vi "CAEN-PSM_1471.vi"() -> ()   [LabVIEW 2018]
doc: "This example shows how to configure the instrument's output voltage level, over current protection, and over voltage protection. The actual voltage level and actual current level are returned as well as whether over voltage protection (OVP) or over current protection (OCP) has been tripped."
uses:
  <vilib>/Utility/file.llb/Write To Spreadsheet File (string).vi
  <instrlib>/CAEN PSM/CAEN PSM.lvlib
panel:
  in  "Stop 1":bool
  in  "Tab Control":T1(tab)
  in  "Set":string[][](table)=[["", "", "", "", "", ""], ["", "", "", "", "", ""], ["", "", "", "", "", ""], ["", "", "", "", "", ""], ["", "", "", "", "", ""], ["", "", "", "", "", ""]]
  out "Monitor":string[][](table)
  in  "Ch (On/Off)":bool[](array[boolean])=[FALSE, FALSE, FALSE, FALSE, FALSE, FALSE, FALSE, FALSE]
  in  "Stop":bool
  in  "Comunication Port":refnum<visa-resource-name>="COM4"
  out "Channel Status":T2(array[cluster])
  in  "File name":string="Name"
  in  "Save":bool
  in  "Grid on/off":enum32{"Radio Selection 1", "Radio Selection 2"}(radio)=enum."Radio Selection 2"
  out "I CH0":T3(graph)
  out "V CH0":T4(graph)
  out "V Ch1":T4(graph)
  out "I CH1":T3(graph)
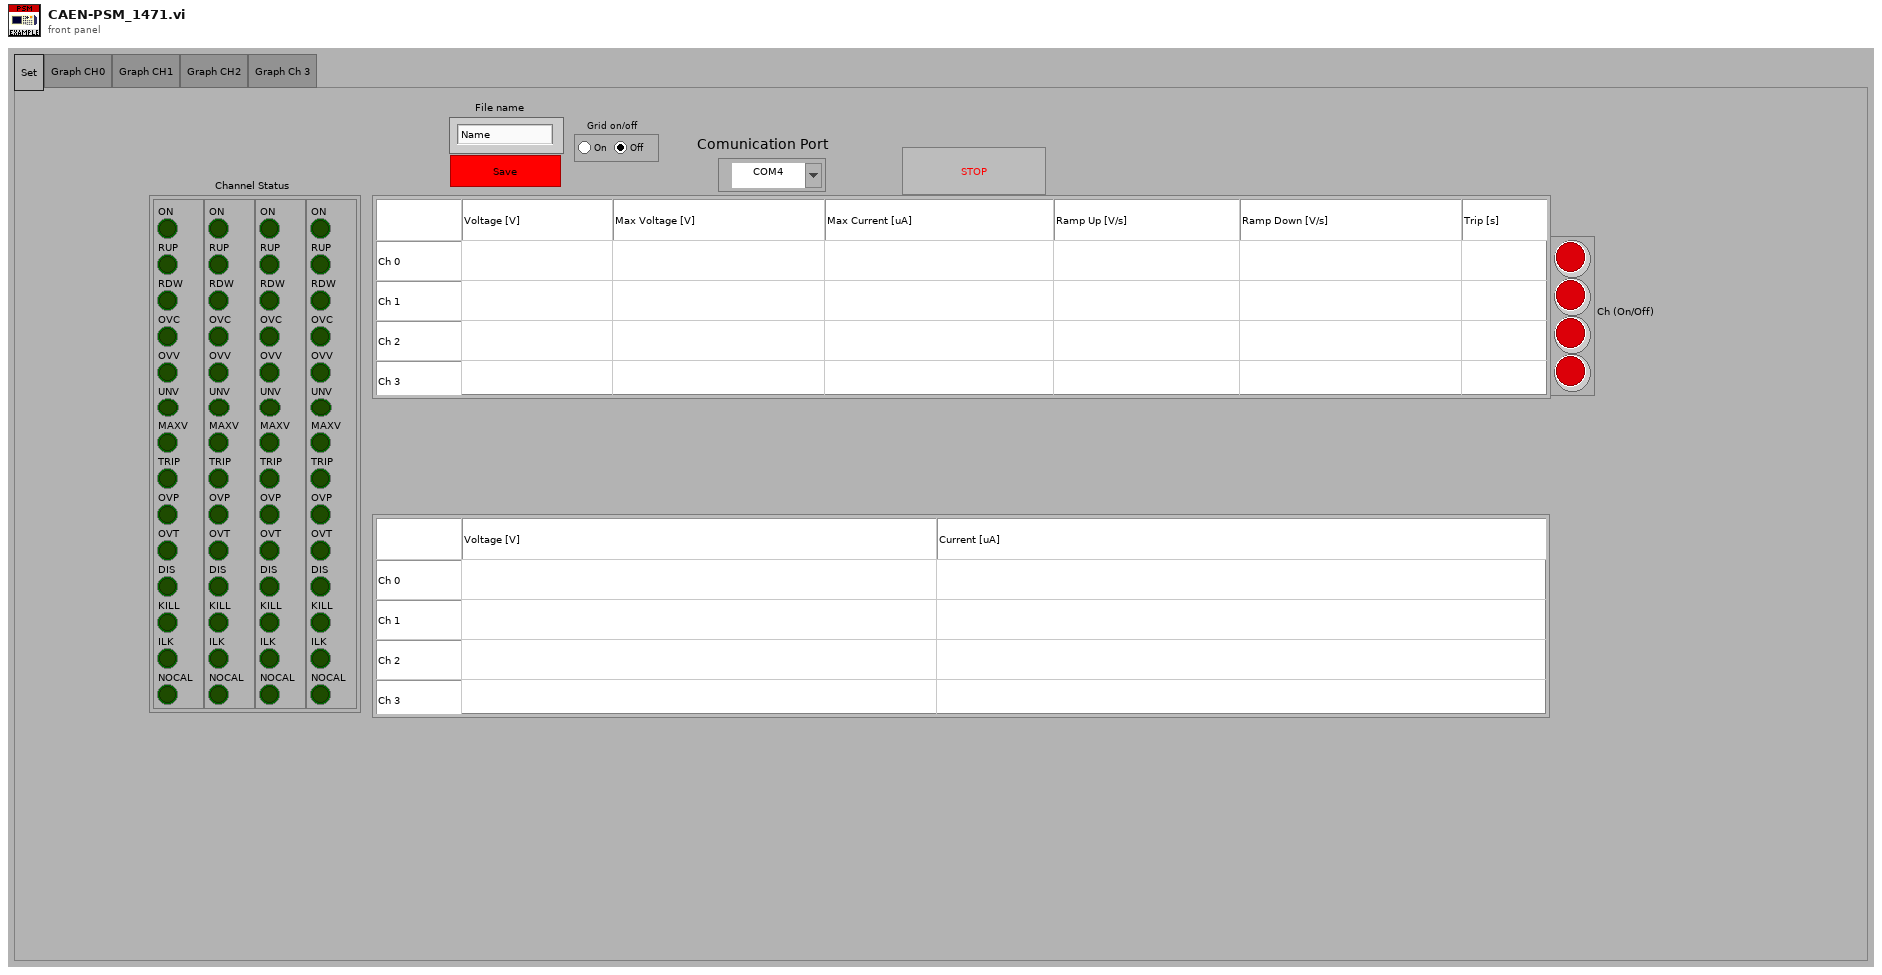
[diagram p1: front panel]
types:
  T1 = enum32{"Set", "Graph CH0", "Graph CH1", "Graph CH2", "Graph Ch 3"}
  T2 = cluster{"ON":bool, "RUP":bool, "RDW":bool, "OVC":bool, "OVV":bool, "UNV":bool, "MAXV":bool, "TRIP":bool, "OVP":bool, "OVT":bool, "DIS":bool, "KILL":bool, "ILK":bool, "NOCAL":bool}[]
  T3 = cluster{"seconds since 1Jan1904":timestamp, "IMon value":dbl}[]
  T4 = cluster{"seconds since 1Jan1904":timestamp, "VMon value":dbl}[]
  T5 = cluster{"Baud Rate":u32, "Parity":u16, "Data Bits":u16, "Stop Bits":u16, "Flow Control":u16}
  T6 = typedef "CAEN PSM.lvlib/BoardHandle.ctl" = cluster{"VISA resource name":refnum<visa-resource-name>, "Board address":u8, "NChannels":u8}
  T7 = cluster{"ON":bool, "RUP":bool, "RDW":bool, "OVC":bool, "OVV":bool, "UNV":bool, "MAXV":bool, "TRIP":bool, "OVP":bool, "OVT":bool, "DIS":bool, "KILL":bool, "ILK":bool, "NOCAL":bool}
  T8 = cluster{"seconds since 1Jan1904":timestamp, "VMon value":dbl}
  T9 = cluster{"seconds since 1Jan1904":timestamp, "IMon value":dbl}
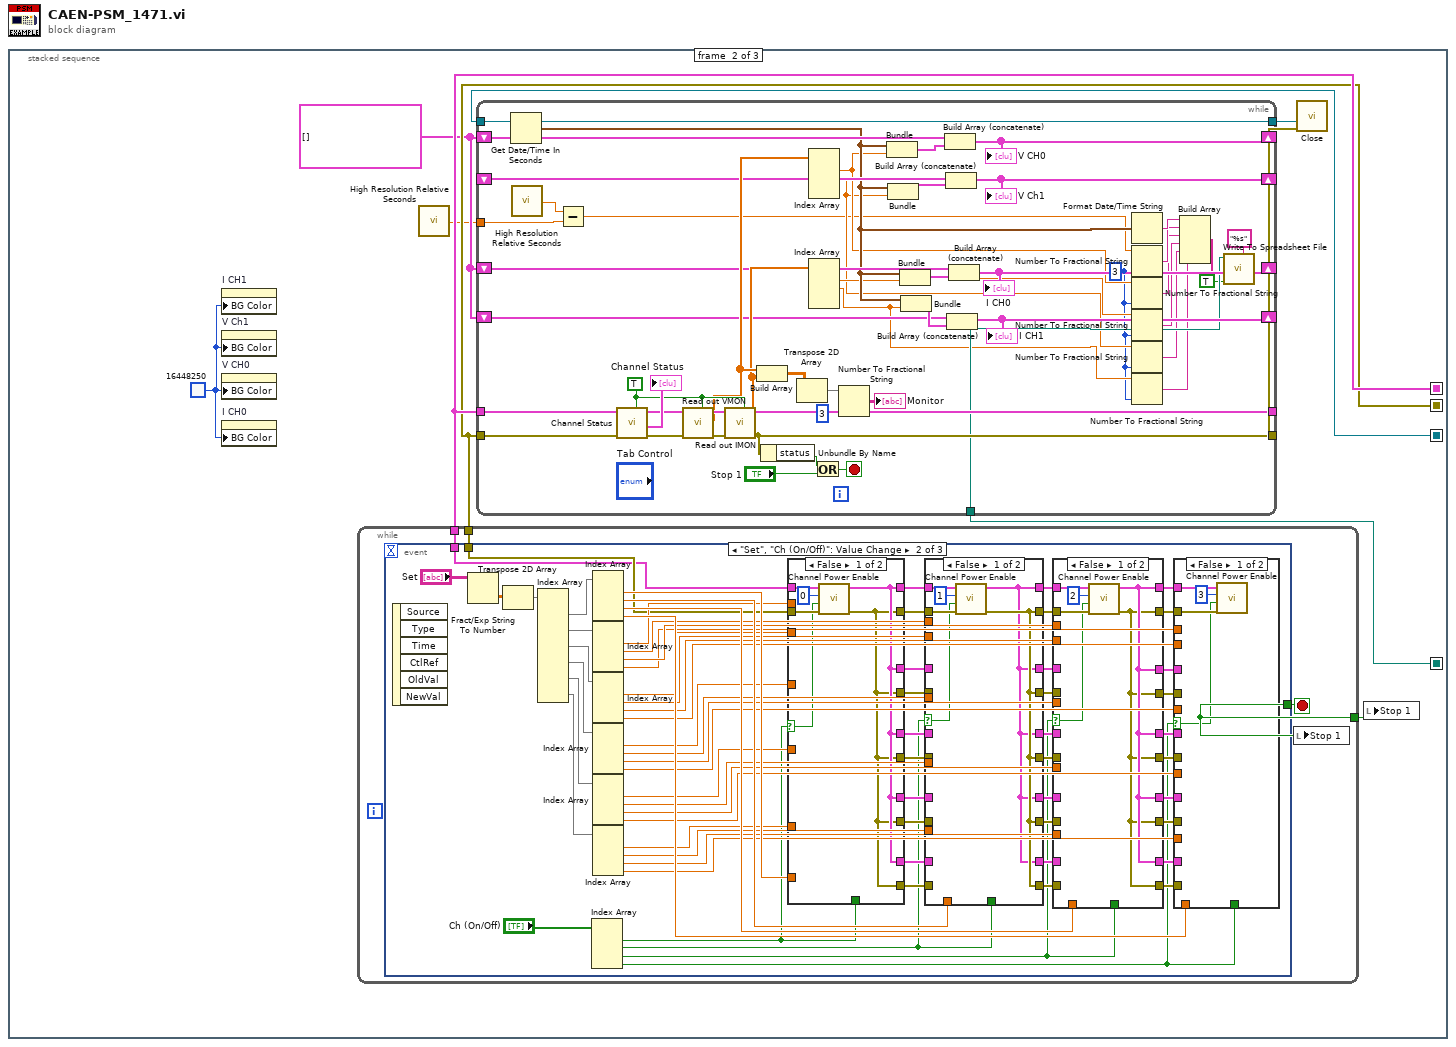
[diagram p0: block diagram]
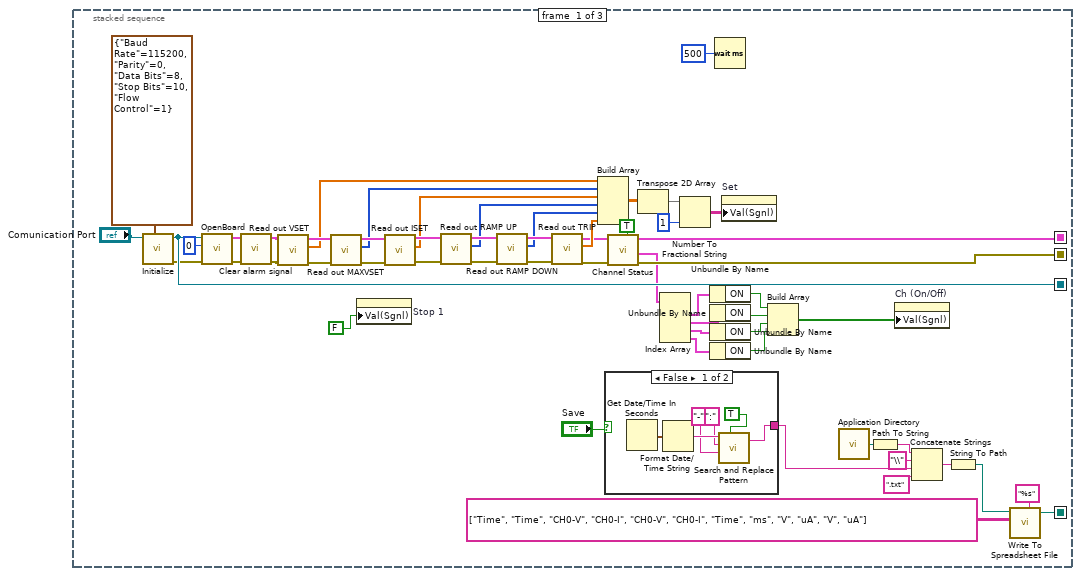
[diagram p2: hidden frame]
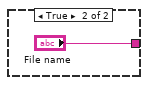
[diagram p3: hidden frame]
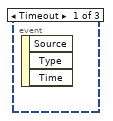
[diagram p4: hidden frame]
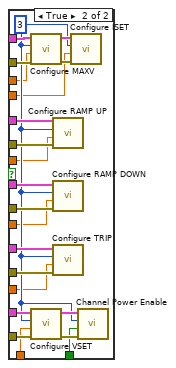
[diagram p5: hidden frame]
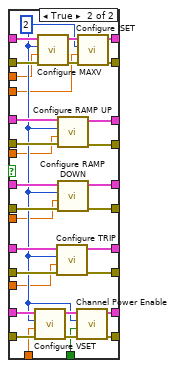
[diagram p6: hidden frame]
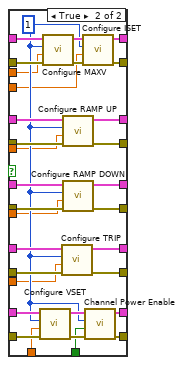
[diagram p7: hidden frame]
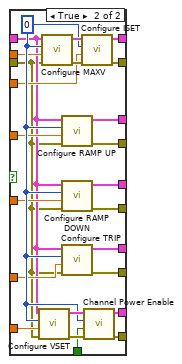
[diagram p8: hidden frame]
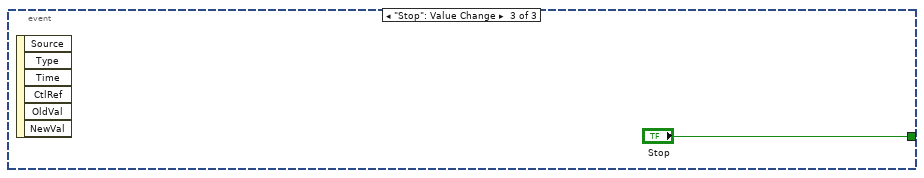
[diagram p9: hidden frame]
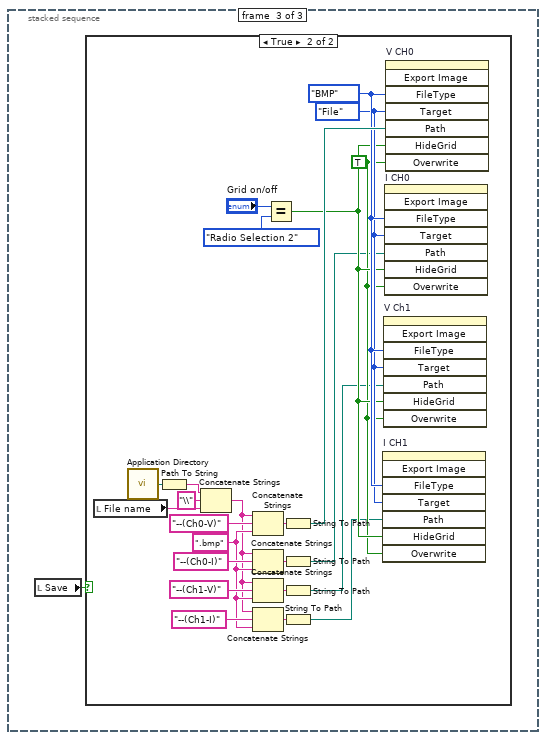
[diagram p10: hidden frame]
diagram:
  n1 = stacked-sequence {
    seq-local: [w56 _ _] -> [_ w71 _]
    seq-local: [w55 _ _] -> [_ w70 _]
    seq-local: [w57 _ _] -> [_ w74 _]
    seq-local: [w11 _ _] -> [_ w66 _]
    frame #0 {
      n2 = call <instrlib>:"Initialize.vi"("Serial Configuration"=T5 {"Baud Rate"=115200, "Parity"=0, "Data Bits"=8, "Stop Bits"=10, "Flow Control"=1}, "VISA resource name"="Comunication Port") -> ("error out"=w53:errorcluster, "VISA resource name out"=w57:refnum<visa-resource-name>)  [unwired: 8 in]
      n3 = call <instrlib>:"OpenBoard.vi"("error in (no error)"=w53, "Board Address"=u8 0, "VISA resource name"=w57) -> ("error out"=w51:errorcluster, "BoardHandle"=w50:T6)  [unwired: 7 in]
      n4 = call <instrlib>:"Clear alarm signal.vi"("error in (no error)"=w51, "BoardHandle"=w50) -> ("error out"=w37:errorcluster, "BoardHandle out"=w38:T6)  [unwired: 8 in]
      n5 = call <instrlib>:"Read out VSET.vi"("error in (no error)"=w37, "BoardHandle"=w38) -> ("error out"=w47:errorcluster, "Vset values (V)"=w33:dbl[], "BoardHandle out"=w48:T6)  [unwired: 6 in, 1 out]
      n6 = call <instrlib>:"Read out MAXVSET.vi"("error in (no error)"=w47, "BoardHandle"=w48) -> ("error out"=w45:errorcluster, "Voltage max values (V)"=w32:i32[], "BoardHandle out"=w46:T6)  [unwired: 6 in, 1 out]
      n7 = property on="Stop 1" class="Bool (strict)"("Val(Sgnl)"=FALSE ("Value (Signaling)")) -> ()  [unwired: 2 in, 2 out]
      n8 = call <instrlib>:"Read out ISET.vi"("error in (no error)"=w45, "BoardHandle"=w46) -> ("error out"=w43:errorcluster, "ISet values (uA)"=w31:dbl[], "BoardHandle out"=w44:T6)  [unwired: 6 in, 1 out]
      n9 = call <instrlib>:"Read out RAMP UP.vi"("error in (no error)"=w43, "BoardHandle"=w44) -> ("error out"=w41:errorcluster, "Ramp up values  (V/s)"=w30:i32[], "BoardHandle out"=w42:T6)  [unwired: 6 in, 1 out]
      n10 = call <instrlib>:"Read out RAMP DOWN.vi"("error in (no error)"=w41, "BoardHandle"=w42) -> ("error out"=w39:errorcluster, "Ramp down values  (V/s)"=w29:i32[], "BoardHandle out"=w40:T6)  [unwired: 6 in, 1 out]
      n11 = call <instrlib>:"Read out TRIP.vi"("error in (no error)"=w39, "BoardHandle"=w40) -> ("error out"=w24:errorcluster, "Trip values (s)"=w28:dbl[], "BoardHandle out"=w25:T6)  [unwired: 6 in, 1 out]
      n12 = Build Array(w33, w32, w31, w30, w29, w28) -> (w36:dbl[][])
      n13 = case shown="False" "Save" {
        tunnel: [w58 "File name"] -> w1
        frame False {
          n14 = Get Date/Time In Seconds() -> (seconds since 1Jan1904=w63:timestamp)
          n15 = Format Date/Time String(seconds (now)=w63) -> (date/time string=w62:string)  [unwired: 2 in]
          n16 = call <vilib>:"Search and Replace Pattern.vi"("string"=w62, "regular expression (\"\")"=":" ("regular expression (\"\")"), "replace string (\"\")"="-" ("replace string (\"\")"), "replace all? (F)"=TRUE) -> ("result string"=w58:string)  [unwired: 1 in, 1 out]
        }
        frame True {
        }
      }
      n17 = call <instrlib>:"Channel Status.vi"("All Channels (T)"=TRUE, "error in (no error)"=w24, "BoardHandle"=w25) -> ("error out"=w55:errorcluster, "Channel Status Array"=w23:T2, "BoardHandle out"=w56:T6)  [unwired: 6 in]
      n18 = Transpose 2D Array(2D array=w36) -> (transposed array=w35:dbl[][])
      n19 = Index Array(array=w23) -> (element #1=w22:T7, element #2=w21:T7, element #3=w20:T7, element #4=w19:T7)  [unwired: 4 in]
      n20 = Number To Fractional String(number=w35, precision (6)=i16 1) -> (F-format string=w27:string[][])  [unwired: 2 in]
      n21 = Unbundle By Name(w22) -> ("ON"=w18:bool)
      n22 = Unbundle By Name(w21) -> ("ON"=w17:bool)
      n23 = Unbundle By Name(w20) -> ("ON"=w16:bool)
      n24 = Unbundle By Name(w19) -> ("ON"=w15:bool)
      n25 = Wait (ms)(milliseconds to wait=u32 500) -> ()  [unwired: 1 out]
      n26 = property on="Set" class="Tbl (strict)"("Val(Sgnl)"=w27) -> ()  [unwired: 2 in, 2 out]
      n27 = Build Array(w18, w17, w16, w15) -> (w14:bool[])
      n28 = call <vilib>:"Application Directory.vi"() -> ("Application Directory"=w5:path)
      n29 = Path To String(path=w5) -> (string=w4:string)
      n30 = property on="Ch (On/Off)" class="Arr (strict)"("Val(Sgnl)"=w14) -> ()  [unwired: 2 in, 2 out]
      n31 = Concatenate Strings(w4, "\\" ("string"), w1, ".txt" ("string")) -> (w9:string)
      n32 = String To Path(string=w9) -> (path=w10:path)
      n33 = call-poly <vilib>:"Write To Spreadsheet File.vi"("format (%s)"="%s", "2D data"=string[][] [["Time", "Time", "CH0-V", "CH0-I", "CH0-V", "CH0-I"], ["Time", "ms", "V", "uA", "V", "uA"]], "file path (dialog if empty)"=w10) -> ("new file path (Not A Path if cancelled)"=w11:path)  [unwired: 5 in]
    }
    frame #1 {
      w67 = u32 16448250
      w68 = T4 []
      n34 = property on="I CH1" class="XYGraph (strict)"("BG Color"=w67) -> ()  [unwired: 2 in, 2 out]
      n35 = property on="V Ch1" class="XYGraph (strict)"("BG Color"=w67) -> ()  [unwired: 2 in, 2 out]
      n36 = property on="V CH0" class="XYGraph (strict)"("BG Color"=w67) -> ()  [unwired: 2 in, 2 out]
      n37 = property on="I CH0" class="XYGraph (strict)"("BG Color"=w67) -> ()  [unwired: 2 in, 2 out]
      n38 = while {
        tunnel: w71 -> [w77]
        tunnel: w70 -> [w76]
        tunnel: [w75] -> w69
        stop <- w75 stop-if-true
        n39 = event shown="[1] \"Set\", \"Ch (On/Off)\": Value Change" {
          selector: _ -> [_ _ _]
          dyn-events: _ -> [_ _ _]
          timeout: _ -> [_ _ _]
          tunnel: [_ _ "Stop"] -> w75
          tunnel: w77 -> [_ w82 _]
          tunnel: w76 -> [_ w83 _]
          event Timeout {
            n40 = event-data() -> ()  [unwired: 1 in, 3 out]
          }
          event "Set", "Ch (On/Off)": Value Change {
            n41 = event-data() -> ()  [unwired: 1 in, 6 out]
            n42 = Fract/Exp String To Number(string="Set") -> (number=w117:dbl[][])  [unwired: 3 in, 1 out]
            n43 = Transpose 2D Array(2D array=w117) -> (transposed array=w116:dbl[][])
            n44 = Index Array(array=w116) -> (element #1=w115:dbl[], element #2=w114:dbl[], element #3=w113:dbl[], element #4=w112:dbl[], element #5=w111:dbl[], element #6=w110:dbl[])  [unwired: 12 in]
            n45 = Index Array(array="Ch (On/Off)") -> (element #1=w81:bool, element #2=w80:bool, element #3=w79:bool, element #4=w78:bool)  [unwired: 4 in]
            n46 = Index Array(array=w115) -> (element #1=w109:dbl, element #2=w108:dbl, element #3=w107:dbl, element #4=w106:dbl)  [unwired: 4 in]
            n47 = Index Array(array=w114) -> (element #1=w105:dbl, element #2=w104:dbl, element #3=w103:dbl, element #4=w102:dbl)  [unwired: 4 in]
            n48 = Index Array(array=w113) -> (element #1=w101:dbl, element #2=w100:dbl, element #3=w99:dbl, element #4=w98:dbl)  [unwired: 4 in]
            n49 = Index Array(array=w112) -> (element #1=w97:dbl, element #2=w96:dbl, element #3=w95:dbl, element #4=w94:dbl)  [unwired: 4 in]
            n50 = Index Array(array=w111) -> (element #1=w93:dbl, element #2=w92:dbl, element #3=w91:dbl, element #4=w90:dbl)  [unwired: 4 in]
            n51 = Index Array(array=w110) -> (element #1=w89:dbl, element #2=w88:dbl, element #3=w87:dbl, element #4=w86:dbl)  [unwired: 4 in]
            n52 = case shown="False" w81 {
              selector: w81 -> [w250 _]
              tunnel: [w252 w277] -> w147
              tunnel: [w254 w276] -> w146
              tunnel: [w252 w275] -> w141
              tunnel: [w254 w274] -> w140
              tunnel: [w254 w273] -> w135
              tunnel: [w252 w272] -> w130
              tunnel: [w254 w271] -> w129
              tunnel: [w252 w270] -> w124
              tunnel: [w252 w267] -> w123
              tunnel: [w254 w266] -> w122
              tunnel: w109 -> [_ w264]
              tunnel: w81 -> [_ w263]
              tunnel: w105 -> [_ w262]
              tunnel: w101 -> [_ w261]
              tunnel: w97 -> [_ w260]
              tunnel: w93 -> [_ w259]
              tunnel: w89 -> [_ w258]
              tunnel: w83 -> [w253 w256]
              tunnel: w82 -> [w255 w257]
              frame False {
                n53 = call <instrlib>:"Channel Power Enable.vi"("error in (no error)"=w253, "Enable (OFF)"=w250, "Channel (0)"=u8 0, "BoardHandle"=w255) -> ("error out"=w252:errorcluster, "BoardHandle out"=w254:T6)  [unwired: 6 in]
              }
              frame True {
                w265 = u8 0 ("Channel (0)")
                n54 = call <instrlib>:"Configure VSET.vi"("error in (no error)"=w256, "Voltage Level (0.0 V)"=w264, "Channel (0)"=w265, "BoardHandle"=w257) -> ("error out"=w269:errorcluster, "BoardHandle out"=w268:T6)  [unwired: 6 in]
                n55 = call <instrlib>:"Configure MAXV.vi"("error in (no error)"=w256, "Voltage Max (0.0 V)"=w262, "Channel (0)"=w265, "BoardHandle"=w257) -> ("error out"=w278:errorcluster, "BoardHandle out"=w279:T6)  [unwired: 6 in]
                n56 = call <instrlib>:"Configure RAMP UP.vi"("error in (no error)"=w256, "Voltage ramp up (0 V/s)"=w260, "Channel (0)"=w265, "BoardHandle"=w257) -> ("error out"=w275:errorcluster, "BoardHandle out"=w274:T6)  [unwired: 6 in]
                n57 = call <instrlib>:"Configure RAMP DOWN.vi"("error in (no error)"=w256, "Voltage ramp down (0 V/s)"=w259, "Channel (0)"=w265, "BoardHandle"=w257) -> ("error out"=w272:errorcluster, "BoardHandle out"=w273:T6)  [unwired: 6 in]
                n58 = call <instrlib>:"Configure TRIP.vi"("error in (no error)"=w256, "Trip (0.00 s)"=w258, "Channel (0)"=w265, "BoardHandle"=w257) -> ("error out"=w270:errorcluster, "BoardHandle out"=w271:T6)  [unwired: 6 in]
                n59 = call <instrlib>:"Configure ISET.vi"("error in (no error)"=w278, "Current Limit (0.00 uA)"=w261, "Channel (0)"=w265, "BoardHandle"=w279) -> ("error out"=w277:errorcluster, "BoardHandle out"=w276:T6)  [unwired: 6 in]
                n60 = call <instrlib>:"Channel Power Enable.vi"("error in (no error)"=w269, "Enable (OFF)"=w263, "Channel (0)"=w265, "BoardHandle"=w268) -> ("error out"=w267:errorcluster, "BoardHandle out"=w266:T6)  [unwired: 6 in]
              }
            }
            n61 = case shown="False" w80 {
              selector: w80 -> [w212 _]
              tunnel: w147 -> [w216 w247]
              tunnel: w146 -> [w217 w246]
              tunnel: [w214 w245] -> w145
              tunnel: [w215 w244] -> w144
              tunnel: w141 -> [_ w243]
              tunnel: w140 -> [_ w242]
              tunnel: [w215 w241] -> w139
              tunnel: [w214 w240] -> w138
              tunnel: w135 -> [_ w239]
              tunnel: [w214 w238] -> w134
              tunnel: [w215 w237] -> w131
              tunnel: w130 -> [_ w236]
              tunnel: w129 -> [_ w235]
              tunnel: [w214 w234] -> w128
              tunnel: [w215 w233] -> w125
              tunnel: w124 -> [_ w232]
              tunnel: w123 -> [_ w229]
              tunnel: w122 -> [_ w228]
              tunnel: [w214 w227] -> w119
              tunnel: [w215 w226] -> w118
              tunnel: w108 -> [_ w224]
              tunnel: w80 -> [_ w223]
              tunnel: w104 -> [_ w222]
              tunnel: w100 -> [_ w221]
              tunnel: w96 -> [_ w220]
              tunnel: w92 -> [_ w219]
              tunnel: w88 -> [_ w218]
              frame False {
                n62 = call <instrlib>:"Channel Power Enable.vi"("error in (no error)"=w216, "Enable (OFF)"=w212, "Channel (0)"=u8 1, "BoardHandle"=w217) -> ("error out"=w215:errorcluster, "BoardHandle out"=w214:T6)  [unwired: 6 in]
              }
              frame True {
                w225 = u8 1 ("Channel (0)")
                n63 = call <instrlib>:"Configure VSET.vi"("error in (no error)"=w229, "Voltage Level (0.0 V)"=w224, "Channel (0)"=w225, "BoardHandle"=w228) -> ("error out"=w230:errorcluster, "BoardHandle out"=w231:T6)  [unwired: 6 in]
                n64 = call <instrlib>:"Configure MAXV.vi"("error in (no error)"=w247, "Voltage Max (0.0 V)"=w222, "Channel (0)"=w225, "BoardHandle"=w246) -> ("error out"=w249:errorcluster, "BoardHandle out"=w248:T6)  [unwired: 6 in]
                n65 = call <instrlib>:"Configure TRIP.vi"("error in (no error)"=w232, "Trip (0.00 s)"=w218, "Channel (0)"=w225, "BoardHandle"=w235) -> ("error out"=w233:errorcluster, "BoardHandle out"=w234:T6)  [unwired: 6 in]
                n66 = call <instrlib>:"Configure RAMP UP.vi"("error in (no error)"=w243, "Voltage ramp up (0 V/s)"=w220, "Channel (0)"=w225, "BoardHandle"=w242) -> ("error out"=w241:errorcluster, "BoardHandle out"=w240:T6)  [unwired: 6 in]
                n67 = call <instrlib>:"Configure RAMP DOWN.vi"("error in (no error)"=w236, "Voltage ramp down (0 V/s)"=w219, "Channel (0)"=w225, "BoardHandle"=w239) -> ("error out"=w237:errorcluster, "BoardHandle out"=w238:T6)  [unwired: 6 in]
                n68 = call <instrlib>:"Configure ISET.vi"("error in (no error)"=w249, "Current Limit (0.00 uA)"=w221, "Channel (0)"=w225, "BoardHandle"=w248) -> ("error out"=w244:errorcluster, "BoardHandle out"=w245:T6)  [unwired: 6 in]
                n69 = call <instrlib>:"Channel Power Enable.vi"("error in (no error)"=w230, "Enable (OFF)"=w223, "Channel (0)"=w225, "BoardHandle"=w231) -> ("error out"=w226:errorcluster, "BoardHandle out"=w227:T6)  [unwired: 6 in]
              }
            }
            n70 = case shown="False" w79 {
              selector: w79 -> [w176 _]
              tunnel: w145 -> [w178 w209]
              tunnel: w144 -> [w179 w208]
              tunnel: [w175 w207] -> w143
              tunnel: [w174 w206] -> w142
              tunnel: w139 -> [_ w205]
              tunnel: w138 -> [_ w204]
              tunnel: [w174 w203] -> w137
              tunnel: [w175 w202] -> w136
              tunnel: w134 -> [_ w201]
              tunnel: [w175 w200] -> w133
              tunnel: [w174 w199] -> w132
              tunnel: w131 -> [_ w198]
              tunnel: w128 -> [_ w197]
              tunnel: [w175 w196] -> w127
              tunnel: [w174 w195] -> w126
              tunnel: w125 -> [_ w194]
              tunnel: [w174 w191] -> w121
              tunnel: [w175 w190] -> w120
              tunnel: w119 -> [_ w189]
              tunnel: w118 -> [_ w188]
              tunnel: w107 -> [_ w186]
              tunnel: w79 -> [_ w185]
              tunnel: w103 -> [_ w184]
              tunnel: w99 -> [_ w183]
              tunnel: w95 -> [_ w182]
              tunnel: w91 -> [_ w181]
              tunnel: w87 -> [_ w180]
              frame False {
                n71 = call <instrlib>:"Channel Power Enable.vi"("error in (no error)"=w179, "Enable (OFF)"=w176, "Channel (0)"=u8 2, "BoardHandle"=w178) -> ("error out"=w174:errorcluster, "BoardHandle out"=w175:T6)  [unwired: 6 in]
              }
              frame True {
                w187 = u8 2 ("Channel (0)")
                n72 = call <instrlib>:"Configure VSET.vi"("error in (no error)"=w188, "Voltage Level (0.0 V)"=w186, "Channel (0)"=w187, "BoardHandle"=w189) -> ("error out"=w192:errorcluster, "BoardHandle out"=w193:T6)  [unwired: 6 in]
                n73 = call <instrlib>:"Configure MAXV.vi"("error in (no error)"=w208, "Voltage Max (0.0 V)"=w184, "Channel (0)"=w187, "BoardHandle"=w209) -> ("error out"=w211:errorcluster, "BoardHandle out"=w210:T6)  [unwired: 6 in]
                n74 = call <instrlib>:"Configure TRIP.vi"("error in (no error)"=w194, "Trip (0.00 s)"=w180, "Channel (0)"=w187, "BoardHandle"=w197) -> ("error out"=w195:errorcluster, "BoardHandle out"=w196:T6)  [unwired: 6 in]
                n75 = call <instrlib>:"Configure RAMP UP.vi"("error in (no error)"=w205, "Voltage ramp up (0 V/s)"=w182, "Channel (0)"=w187, "BoardHandle"=w204) -> ("error out"=w203:errorcluster, "BoardHandle out"=w202:T6)  [unwired: 6 in]
                n76 = call <instrlib>:"Configure RAMP DOWN.vi"("error in (no error)"=w198, "Voltage ramp down (0 V/s)"=w181, "Channel (0)"=w187, "BoardHandle"=w201) -> ("error out"=w199:errorcluster, "BoardHandle out"=w200:T6)  [unwired: 6 in]
                n77 = call <instrlib>:"Channel Power Enable.vi"("error in (no error)"=w192, "Enable (OFF)"=w185, "Channel (0)"=w187, "BoardHandle"=w193) -> ("error out"=w191:errorcluster, "BoardHandle out"=w190:T6)  [unwired: 6 in]
                n78 = call <instrlib>:"Configure ISET.vi"("error in (no error)"=w211, "Current Limit (0.00 uA)"=w183, "Channel (0)"=w187, "BoardHandle"=w210) -> ("error out"=w206:errorcluster, "BoardHandle out"=w207:T6)  [unwired: 6 in]
              }
            }
            n79 = case shown="False" w78 {
              selector: w78 -> [w149 _]
              tunnel: w143 -> [w151 w171]
              tunnel: w142 -> [w150 w170]
              tunnel: w137 -> [_ w169]
              tunnel: w136 -> [_ w168]
              tunnel: w133 -> [_ w167]
              tunnel: w132 -> [_ w166]
              tunnel: w127 -> [_ w165]
              tunnel: w126 -> [_ w164]
              tunnel: w121 -> [_ w162]
              tunnel: w120 -> [_ w161]
              tunnel: w106 -> [_ w158]
              tunnel: w78 -> [_ w157]
              tunnel: w102 -> [_ w156]
              tunnel: w98 -> [_ w155]
              tunnel: w94 -> [_ w154]
              tunnel: w90 -> [_ w153]
              tunnel: w86 -> [_ w152]
              frame False {
                n80 = call <instrlib>:"Channel Power Enable.vi"("error in (no error)"=w150, "Enable (OFF)"=w149, "Channel (0)"=u8 3, "BoardHandle"=w151) -> ()  [unwired: 6 in, 2 out]
              }
              frame True {
                w159 = u8 3 ("Channel (0)")
                n81 = call <instrlib>:"Configure MAXV.vi"("error in (no error)"=w170, "Voltage Max (0.0 V)"=w156, "Channel (0)"=w159, "BoardHandle"=w171) -> ("error out"=w172:errorcluster, "BoardHandle out"=w173:T6)  [unwired: 6 in]
                n82 = call <instrlib>:"Configure VSET.vi"("error in (no error)"=w162, "Voltage Level (0.0 V)"=w158, "Channel (0)"=w159, "BoardHandle"=w161) -> ("error out"=w163:errorcluster, "BoardHandle out"=w160:T6)  [unwired: 6 in]
                n83 = call <instrlib>:"Configure RAMP UP.vi"("error in (no error)"=w169, "Voltage ramp up (0 V/s)"=w154, "Channel (0)"=w159, "BoardHandle"=w168) -> ()  [unwired: 6 in, 2 out]
                n84 = call <instrlib>:"Configure RAMP DOWN.vi"("error in (no error)"=w166, "Voltage ramp down (0 V/s)"=w153, "Channel (0)"=w159, "BoardHandle"=w167) -> ()  [unwired: 6 in, 2 out]
                n85 = call <instrlib>:"Configure TRIP.vi"("error in (no error)"=w164, "Trip (0.00 s)"=w152, "Channel (0)"=w159, "BoardHandle"=w165) -> ()  [unwired: 6 in, 2 out]
                n86 = call <instrlib>:"Configure ISET.vi"("error in (no error)"=w172, "Current Limit (0.00 uA)"=w155, "Channel (0)"=w159, "BoardHandle"=w173) -> ()  [unwired: 6 in, 2 out]
                n87 = call <instrlib>:"Channel Power Enable.vi"("error in (no error)"=w163, "Enable (OFF)"=w157, "Channel (0)"=w159, "BoardHandle"=w160) -> ()  [unwired: 6 in, 2 out]
              }
            }
          }
          event "Stop": Value Change {
            n88 = event-data() -> ()  [unwired: 1 in, 6 out]
          }
        }
        n89 = local write "Stop 1"(w75) -> ()
      }
      n90 = call <vilib>:"High Resolution Relative Seconds.vi"() -> ("relative seconds"=w65:dbl)
      n91 = while {
        tunnel: [w326] -> _
        tunnel: [w322] -> w73
        tunnel: w71 -> [w321]
        tunnel: w70 -> [w320]
        tunnel: w74 -> [w319]
        tunnel: [w319] -> w72
        shift-right: [w310] -> _
        shift-left: w68 -> [w312]
        shift-right: [w307] -> _
        shift-left: w68 -> [w308]
        shift-right: [w301] -> _
        shift-left: _ -> [w305]
        shift-right: [w300] -> _
        shift-left: w68 -> [w303]
        tunnel: w66 -> [w299]
        tunnel: w65 -> [w292]
        stop <- w325 stop-if-true
        w282 = 3
        w324 = TRUE ("All Channels (T)")
        n92 = Get Date/Time In Seconds() -> (seconds since 1Jan1904=w298:timestamp)
        n93 = call <vilib>:"High Resolution Relative Seconds.vi"() -> ("relative seconds"=w293:dbl)
        n94 = Subtract(x=w293, y=w292) -> (x-y=w291:dbl)
        n95 = call <instrlib>:"Channel Status.vi"("All Channels (T)"=w324, "error in (no error)"=w320, "BoardHandle"=w321) -> ("error out"=w327:errorcluster, "Channel Status Array"=→"Channel Status":T2, "BoardHandle out"=w328:T6)  [unwired: 6 in]
        n96 = call <instrlib>:"Read out VMON.vi"("All Channels (T)"=w324, "error in (no error)"=w327, "BoardHandle"=w328) -> ("error out"=w330:errorcluster, "VMon values (V)"=w315:dbl[], "BoardHandle out"=w329:T6)  [unwired: 6 in]
        n97 = call <instrlib>:"Read out IMON.vi"("All Channels (T)"=w324, "error in (no error)"=w330, "BoardHandle"=w329) -> ("error out"=w322:errorcluster, "IMon values (uA)"=w314:dbl[], "BoardHandle out"=w326:T6)  [unwired: 5 in, 1 out]
        n98 = Build Array(w315, w314) -> (w302:dbl[][])
        n99 = Unbundle By Name(w322) -> ("status"=w323:bool)
        n100 = Transpose 2D Array(2D array=w302) -> (transposed array=w317:dbl[][])
        n101 = Index Array(array=w315) -> (element #1=w297:dbl, element #2=w295:dbl)  [unwired: 4 in, 2 out]
        n102 = Index Array(array=w314) -> (element #1=w296:dbl, element #2=w294:dbl)  [unwired: 4 in, 2 out]
        n103 = Or(x=w323, y="Stop 1") -> (x .or. y?=w325:bool)
        n104 = Number To Fractional String(number=w317, precision (6)=i16 3) -> (F-format string=→"Monitor":string[][])  [unwired: 2 in]
        n105 = Bundle("seconds since 1Jan1904"=w298, "VMon value"=w297) -> (w311:T8)  [unwired: 1 in]
        n106 = Bundle("seconds since 1Jan1904"=w298, "VMon value"=w295) -> (w306:T8)  [unwired: 1 in]
        n107 = Bundle("seconds since 1Jan1904"=w298, "IMon value"=w296) -> (w309:T9)  [unwired: 1 in]
        n108 = Bundle("seconds since 1Jan1904"=w298, "IMon value"=w294) -> (w304:T9)  [unwired: 1 in]
        n109 = Build Array (concatenate)(w312, w311) -> (w310:T4)
        "V CH0" <- w310
        n110 = Build Array (concatenate)(w305, w306) -> (w301:T4)
        "V Ch1" <- w301
        n111 = Build Array (concatenate)(w303, w304) -> (w300:T3)
        "I CH1" <- w300
        n112 = Build Array (concatenate)(w308, w309) -> (w307:T3)
        "I CH0" <- w307
        n113 = Format Date/Time String(seconds (now)=w298) -> (date/time string=w289:string)  [unwired: 2 in]
        n114 = Number To Fractional String(number=w291, precision (6)=w282) -> (F-format string=w288:string)  [unwired: 2 in]
        n115 = Number To Fractional String(number=w297, precision (6)=w282) -> (F-format string=w285:string)  [unwired: 2 in]
        n116 = Number To Fractional String(number=w296, precision (6)=w282) -> (F-format string=w284:string)  [unwired: 2 in]
        n117 = Number To Fractional String(number=w295, precision (6)=w282) -> (F-format string=w283:string)  [unwired: 2 in]
        n118 = Number To Fractional String(number=w294, precision (6)=w282) -> (F-format string=w281:string)  [unwired: 2 in]
        n119 = Build Array(w289, w288, w285, w284, w283, w281) -> (w286:string[])
        n120 = call-poly <vilib>:"Write To Spreadsheet File.vi"("format (%s)"="%s", "append to file? (new file:F)"=TRUE, "1D data"=w286, "file path (dialog if empty)"=w299) -> ()  [unwired: 4 in, 1 out]
      }
      n121 = call <instrlib>:"Close.vi"("error in (no error)"=w73, "VISA resource name"=w72) -> ()  [unwired: 9 in, 1 out]
      n122 = local write "Stop 1"(w69) -> ()
    }
    frame #2 {
      n123 = local read "Save"() -> (w332:bool)
      n124 = case shown="True" w332 {
        frame False {
        }
        frame True {
          w343 = ".bmp" ("string")
          w339 = enum32{"BMP", "EPS", "EMF", "PICT"}."BMP" ("File Type")
          w338 = enum32{"File", "Clipboard"}."File" ("Target")
          w336 = TRUE ("Hide Grid")
          n125 = local read "File name"() -> (w341:string)
          n126 = call <vilib>:"Application Directory.vi"() -> ("Application Directory"=w355:path)
          n127 = Path To String(path=w355) -> (string=w356:string)
          n128 = Concatenate Strings(w356, "\\" ("string"), w341) -> (w342:string)
          n129 = Concatenate Strings(w342, "--(Ch0-V)" ("string"), w343) -> (w351:string)
          n130 = Concatenate Strings(w342, "--(Ch0-I)" ("string"), w343) -> (w350:string)
          n131 = Concatenate Strings(w342, "--(Ch1-V)" ("string"), w343) -> (w347:string)
          n132 = Concatenate Strings(w342, "--(Ch1-I)" ("string"), w343) -> (w344:string)
          n133 = Equal?(x="Grid on/off", y=enum32{"Radio Selection 1", "Radio Selection 2"}."Radio Selection 2") -> (x = y?=w337:bool)
          n134 = String To Path(string=w351) -> (path=w340:path)
          n135 = String To Path(string=w350) -> (path=w335:path)
          n136 = String To Path(string=w347) -> (path=w334:path)
          n137 = String To Path(string=w344) -> (path=w333:path)
          n138 = invoke on="I CH1" class="XYGraph (strict)" method="Export Image"("FileType"=w339, "Target"=w338, "Path"=w333, "HideGrid"=w337, "Overwrite"=w336) -> ()  [unwired: 3 in, 8 out]
          n139 = invoke on="V Ch1" class="XYGraph (strict)" method="Export Image"("FileType"=w339, "Target"=w338, "Path"=w334, "HideGrid"=w337, "Overwrite"=w336) -> ()  [unwired: 3 in, 8 out]
          n140 = invoke on="I CH0" class="XYGraph (strict)" method="Export Image"("FileType"=w339, "Target"=w338, "Path"=w335, "HideGrid"=w337, "Overwrite"=w336) -> ()  [unwired: 3 in, 8 out]
          n141 = invoke on="V CH0" class="XYGraph (strict)" method="Export Image"("FileType"=w339, "Target"=w338, "Path"=w340, "HideGrid"=w337, "Overwrite"=w336) -> ()  [unwired: 3 in, 8 out]
        }
      }
    }
  }
